vi "AUTOFLIM_AutoScan.vi"(0 "X Scan Center":dbl=55.0, 1 "System#":i16=1, 3 "Mesh":dbl=0.1, 5 "Y Scan Center":dbl=55.0, 7 "Upper thr":dbl=2.0, 9 "Lower Thr":dbl=0.12, 11 "error in (no error)":errorcluster, 12 "X Scan Range":dbl=10.0, 13 "Y Scan Range":dbl=10.0) -> (2 "Xoffset":dbl, 4 "Intensity Graph":dbl[][](array[numeric]), 6 "Nemitters":i32=14, 8 "Yoffset":dbl, 10 "cent":i32[][](array[numeric])=[[44, 6], [40, 23], [42, 24], [52, 29], [12, 42], [52, 42], [24, 45], [80, 48], [52, 57], [7, 76], [17, 76], [32, 80], [86, 88], [53, 94]], 15 "error out":errorcluster)   [LabVIEW 2023]
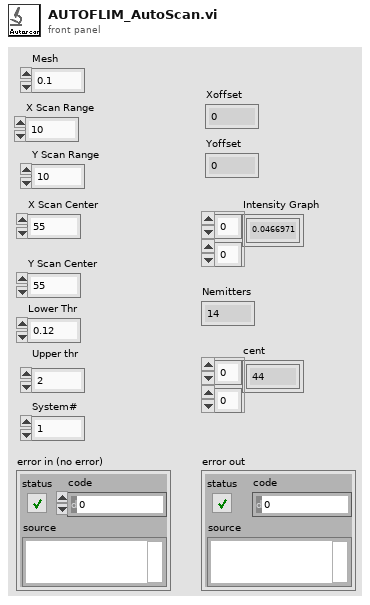
[diagram p1: front panel]
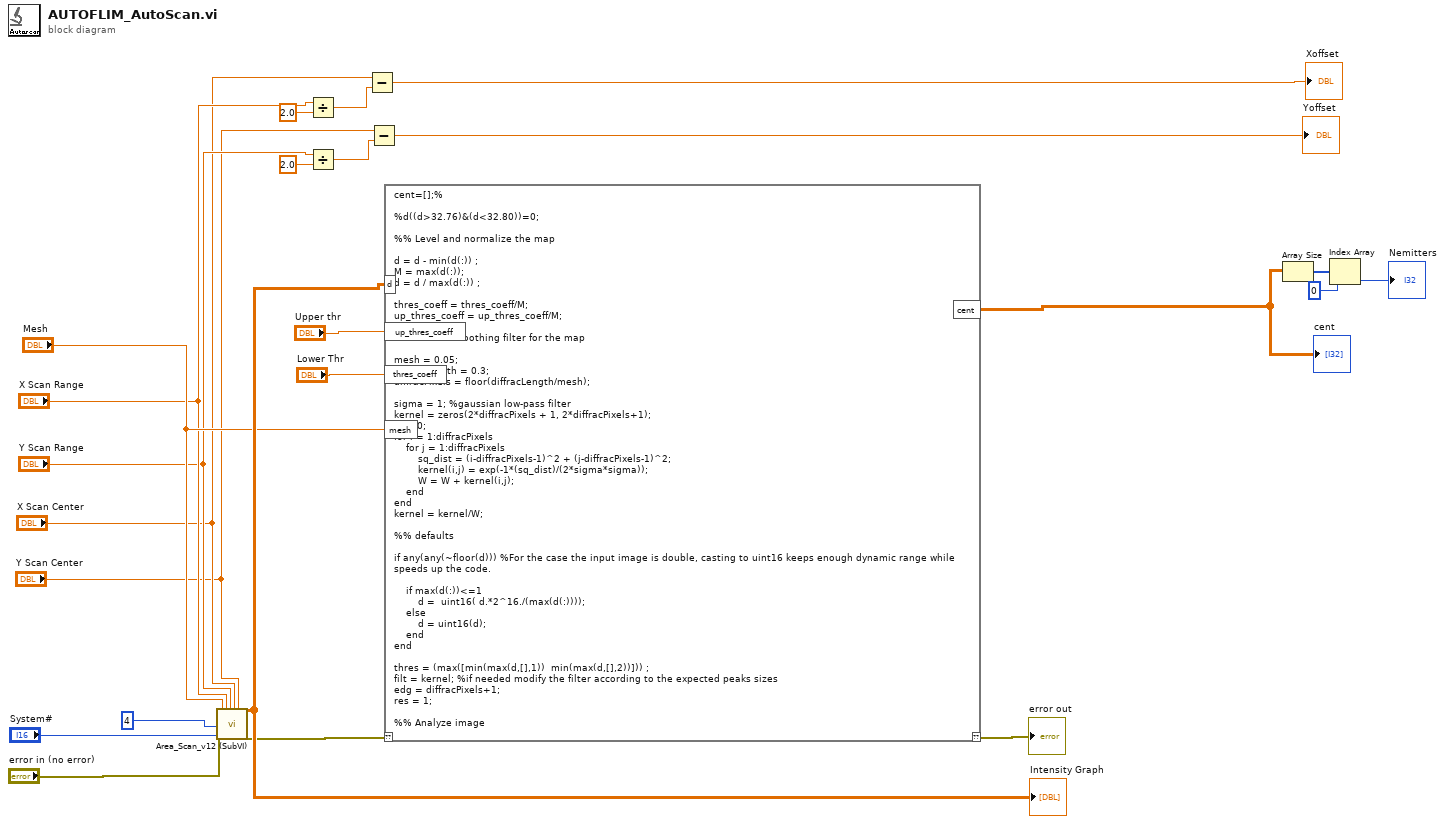
[diagram p0: block diagram]
diagram:
  n1 = call "Area_Scan_v12 (SubVI).vi"("Analog Input"=4, "System no."="System#", "error in (no error)"="error in (no error)", "Mesh in"="Mesh", "X Scan Range"="X Scan Range", "Y Scan Range"="Y Scan Range", "X Scan Center"="X Scan Center", "Y Scan Center"="Y Scan Center") -> ("Intensity Graph"=w14:dbl[][], "error out"=w11:errorcluster)  [unwired: 15 in, 3 out]
  "Intensity Graph" <- w14
  n2 = Divide(x="X Scan Range", y=2.0) -> (x/y=w18:dbl)
  n3 = Divide(x="Y Scan Range", y=2.0) -> (x/y=w17:dbl)
  n4 = Subtract(x="X Scan Center", y=w18) -> (x-y=→"Xoffset":dbl)
  n5 = Subtract(x="Y Scan Center", y=w17) -> (x-y=→"Yoffset":dbl)
  n6 = script code="cent=[];%\n\n%d((d>32.76)&(d<32.80))=0;\n\n%% Level and normalize the map\n\nd = d - min(d(:)) ; \nM = max(d(:));\nd = d / max(d(:)) ;\n\nthres_coeff = thres_coeff/M;\nup_thres_coeff = up_thres_coeff/M;\n\n%% Define smoothing filter for the map\n\nmesh = 0.05;\ndiffracLength = 0.3;\ndiffracPixels = floor(diffracLength/mesh);\n\nsigma = 1; %gaussian low-pass filter\nkernel = zeros(2*diffracPixels + 1, 2*diffracPixels+1);\nW = 0;\nfor i = 1:diffracPixels\n    for j = 1:diffracPixels\n        sq_dist = (i-diffracPixels-1)^2 + (j-diffracPixels-1)^2;\n        kernel(i,j) = exp(-1*(sq_dist)/(2*sigma*sigma));\n        W = W + kernel(i,j);\n    end\nend\nkernel = kernel/W;\n\n%% defaults\n\nif any(any(~floor(d))) %For the case the input image is double, casting to uint16 keeps enough dynamic range while speeds up the code.\n\n    if max(d(:))<=1\n        d =  uint16( d.*2^16./(max(d(:))));\n    else\n        d = uint16(d);\n    end\nend\n\nthres = (max([min(max(d,[],1))  min(max(d,[],2))])) ;\nfilt = kernel; %if needed modify the filter according to the expected peaks sizes\nedg = diffracPixels+1;\nres = 1;\n\n%% Analyze image\n\n\n    \n    % apply threshold\n    if isa(d,'uint8')\n        d=d.*uint8(d>thres);\n    elseif isa(d,'uint16')\n        d=d.*uint16(d>thres);\n    end\n    \n        % smooth image\n        d=conv2(single(d),filt,'same') ;\n        M = max(d(:));\n        thres_coeff = uint16(floor(thres_coeff*M));\n        up_thres_coeff = up_thres_coeff*M;\n        % Apply again threshold (and change if needed according to SNR)\n        d=d.*(d>thres_coeff);\n        \n         bw1 = (d>thres_coeff);\n        CC1 = bwconncomp(bw1);\n              for i = 1:length(CC1.PixelIdxList)\n                      if numel(CC1.PixelIdxList{i}) > (2*diffracPixels)^2\n                           %d(CC1.PixelIdxList{i}) = 0;\n                      end\n               end\n\n        bw2 = (d>thres_coeff/2);\n       CC2 = bwconncomp(bw2);\n              for i = 1:length(CC2.PixelIdxList)\n                      if numel(CC2.PixelIdxList{i}) < 2\n                           %d(CC2.PixelIdxList{i}) = 0;\n                     end\nend\n         \n\n                % switch between local maxima and sub-pixel methods\n            \n                % peak find - using the local maxima approach - 1 pixel resolution\n                \n                % d will be noisy on the edges, and also local maxima looks\n                % for nearest neighbors so edge must be at least 1. We'll skip 'edge' pixels.\n                sd=size(d);\n                [x y]=find(d(edg:sd(1)-edg,edg:sd(2)-edg));\n                \n                % initialize outputs\n \n\n                cent_map=zeros(sd);\n                \n                x=x+edg-1;\n                y=y+edg-1;\n                for j=1:length(y)\n                        if  d(x(j),y(j)) == max(max(d((x(j)- diffracPixels):(x(j)+diffracPixels),(y(j)-diffracPixels):(y(j)+ diffracPixels))))\n\n\n                        if( d(x(j), y(j))< up_thres_coeff)\n                                cent = [cent ;  x(j)  y(j)];\n                        end\n                        %cent_map(x(j),y(j))=cent_map(x(j),y(j))+1; % if a binary matrix output is desired\n                        \n                    end\n                end"("??"=w11, "d"=w14, "up_thres_coeff"="Upper thr", "thres_coeff"="Lower Thr", "mesh"="Mesh") -> ("??"=→"error out":errorcluster, "cent"=w2:dbl[][])
  "cent" <- w2
  n7 = Array Size(array=w2) -> (size(s)=w21:i32[])
  n8 = Index Array(array=w21, index=0) -> (element=→"Nemitters":i32)
